vi "NF WF1973_74 SEQ.vi"(5 "Name(USERNAME)":string="USERNAME", 6 "Read(F)":bool, 7 "Memory No.(0)":i32 min=0 max=128 step=1, 8 "error in (no error)":errorcluster caption="Error IN", 11 "VISAsession":refnum<visa-resource-name>) -> (0 "error out":errorcluster caption="Error OUT", 3 "CopyVISAsession":refnum<visa-resource-name>)   [LabVIEW 2010]
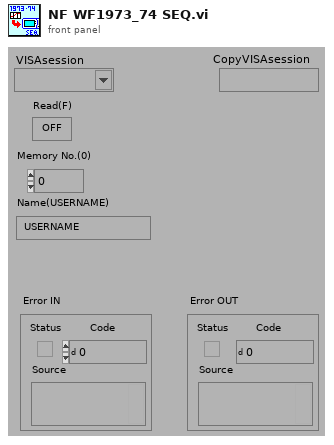
[diagram p1: front panel]
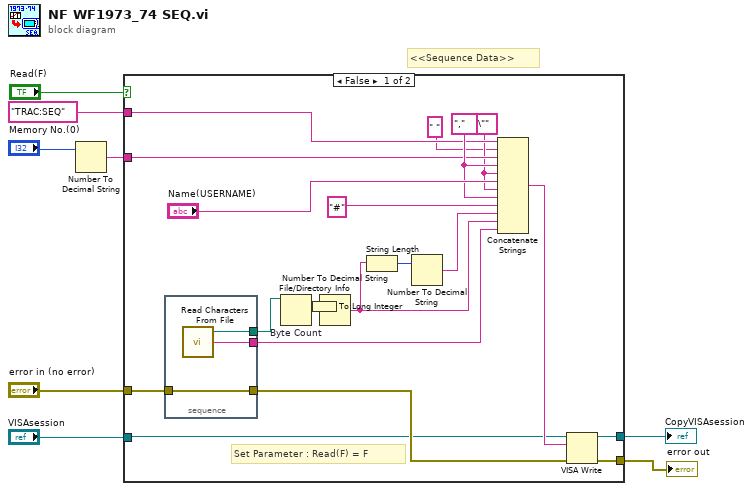
[diagram p0: block diagram]
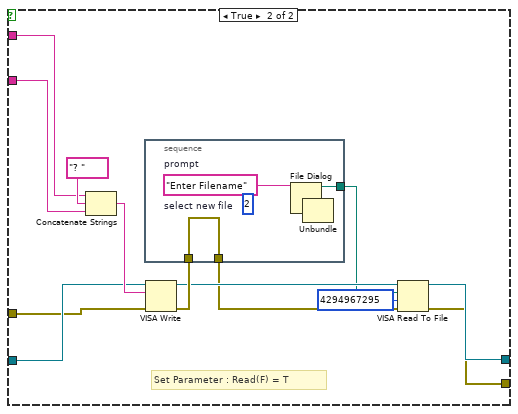
[diagram p2: hidden frame]
diagram:
  # "<<Sequence Data>>"
  n1 = Number To Decimal String(number="Memory No.(0)") -> (decimal integer string=w2:string)  [unwired: 1 in]
  n2 = case shown="FALSE" "Read(F)" {
    tunnel: [w28 w34] -> w8
    tunnel: [w27 w33] -> w7
    tunnel: "TRAC:SEQ" -> [w19 w37]
    tunnel: "error in (no error)" -> [w22 w35]
    tunnel: "VISAsession" -> [w21 w36]
    tunnel: w2 -> [w20 w32]
    frame False {
      w18 = "\""
      w24 = ","
      # "Set Parameter : Read(F) = F"
      n3 = stacked-sequence {
        tunnel: [w31] -> w23
        tunnel: w22 -> [w31]
        tunnel: [w30] -> w14
        tunnel: [w29] -> w11
        frame #0 {
          n4 = call <vilib>:"Read Characters From File.vi"() -> ("new file path (NotAPath if cancelled)"=w29:path, "character string"=w30:string)  [unwired: 6 in, 2 out]
        }
      }
      n5 = File/Directory Info "Byte Count"(path=w11) -> (size=w9:i64)  [unwired: 1 in, 6 out]
      n6 = To Long Integer(number=w9) -> (32bit integer=w16:i32)
      n7 = Number To Decimal String(number=w16) -> (decimal integer string=w10:string)  [unwired: 1 in]
      n8 = String Length(string=w10) -> (length=w13:i32)
      n9 = Number To Decimal String(number=w13) -> (decimal integer string=w12:string)  [unwired: 1 in]
      n10 = Concatenate Strings(w19, " ", w20, w24, w18, "Name(USERNAME)", w18, w24, "#", w12, w10, w14) -> (w25:string)
      n11 = VISA Write(VISA resource name=w21, write buffer=w25, error in (no error)=w23) -> (VISA resource name out=w28:refnum<visa-resource-name>, error out=w27:errorcluster)  [unwired: 1 out]
    }
    frame True {
      # "Set Parameter : Read(F) = T"
      n12 = Concatenate Strings(w37, "? ", w32) -> (w44:string)
      n13 = VISA Write(VISA resource name=w36, write buffer=w44, error in (no error)=w35) -> (VISA resource name out=w41:refnum<visa-resource-name>, error out=w42:errorcluster)  [unwired: 1 out]
      n14 = stacked-sequence {
        tunnel: [w47] -> w38
        tunnel: w42 -> [w46]
        tunnel: [w46] -> w40
        frame #0 {
          w48 = "Enter Filename"  # prompt
          (unwired) i16 2  # select new file
          n15 = File Dialog(7:w48) -> (0:w45:errorcluster, 3:w47:path)  [unwired: 6 in, 2 out]
          n16 = Unbundle(w45) -> ()  [unwired: 3 out]
        }
      }
      n17 = VISA Read To File(8:w40, 9:u32 4294967295 ("カウント (1024)"), 10:w38, 11:w41) -> (0:w33:errorcluster, 3:w34:refnum<visa-resource-name>)  [unwired: 1 out]
    }
  }
  "error out" <- w7
  "CopyVISAsession" <- w8
